vi "CIMAQ_Resample_Proportional.vi"(7 "Interpolation Type":u32(ring) items=["Zero Order", "Bi-Linear", "Quadratic", "Cubic Spline"], 8 "Error In":errorcluster, 9 "YResolution":u32, 10 "X Resolution":u32, 11 "Image In":T1) -> (0 "Error Out":errorcluster, 1 "Y Resolution":i32, 2 "X Resolution":i32, 3 "Image Out":T1)   [LabVIEW 2017]
uses:
  <vilib>/vision/Image Controls.llb/IMAQ Image.ctl
  <vilib>/vision/NI_Vision_Development_Module.lvlib
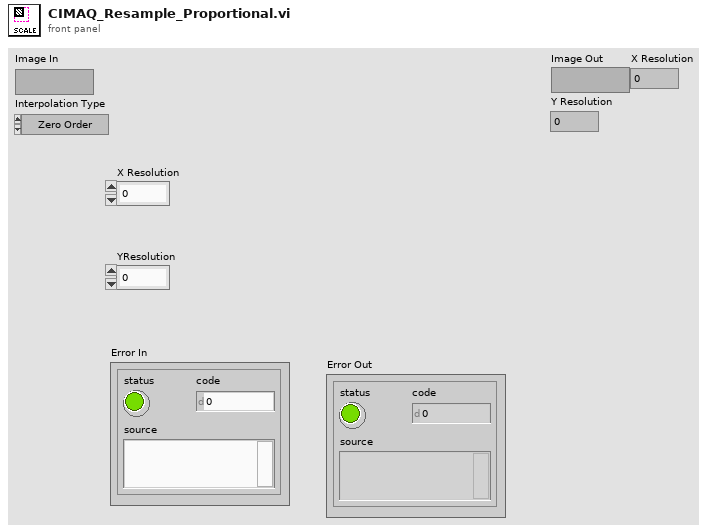
[diagram p1: front panel]
types:
  T1 = typedef "IMAQ Image.ctl" = refnum<image>
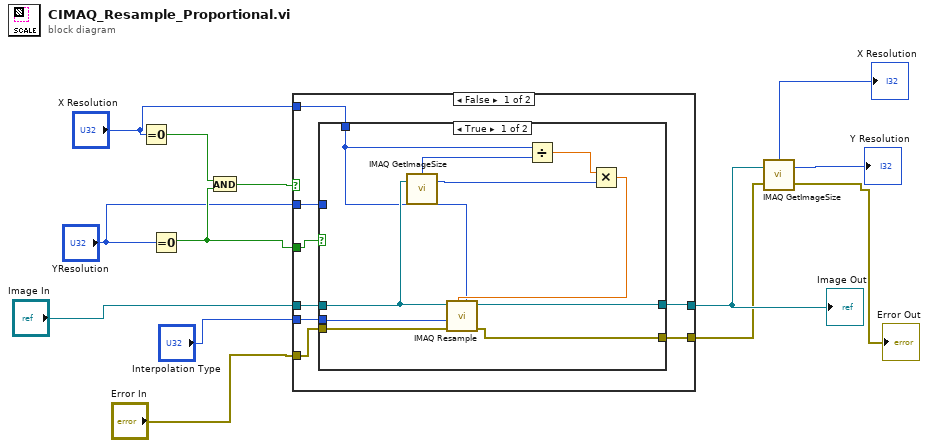
[diagram p0: block diagram]
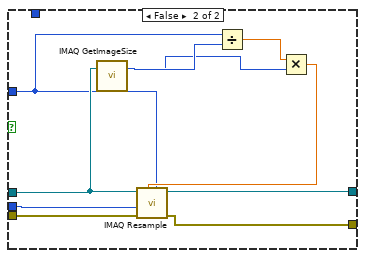
[diagram p2: hidden frame]
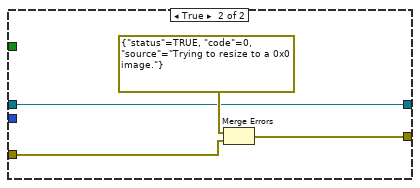
[diagram p3: hidden frame]
diagram:
  n1 = Equal To 0?(x="X Resolution") -> (x = 0?=w12:bool)
  n2 = Equal To 0?(x="YResolution") -> (x = 0?=w9:bool)
  n3 = And(x=w12, y=w9) -> (x .and. y?=w11:bool)
  n4 = case shown="False" w11 {
    tunnel: "Image In" -> [w21 w42]
    tunnel: "Error In" -> [w17 w45]
    tunnel: [w16 w43] -> w3
    tunnel: [w18 w42] -> w6
    tunnel: w9 -> [w20 _]
    tunnel: "X Resolution" -> [w19 _]
    tunnel: "YResolution" -> [w15 _]
    tunnel: "Interpolation Type" -> [w14 _]
    frame False {
      n5 = case shown="True" w20 {
        tunnel: w21 -> [w27 w39]
        tunnel: w19 -> [w26 _]
        tunnel: [w25 w38] -> w18
        tunnel: w17 -> [w24 w37]
        tunnel: [w23 w36] -> w16
        tunnel: w15 -> [_ w35]
        tunnel: w14 -> [w22 w32]
        frame True {
          n6 = call "IMAQ GetImageSize"("Image"=w27) -> ("Y Resolution"=w29:i32, "X Resolution"=w31:i32)  [unwired: 3 in, 1 out]
          n7 = Divide(x=w26, y=w31) -> (x/y=w30:dbl)
          n8 = Multiply(x=w30, y=w29) -> (x*y=w28:dbl)
          n9 = call "IMAQ Resample"("X Resolution"=w26, "Y Resolution"=w28, "error in (no error)"=w24, "Interpolation Type"=w22, "Image Src"=w27) -> ("error out"=w23:errorcluster, "Image Dst Out"=w25:T1)  [unwired: 5 in]
        }
        frame False {
          n10 = call "IMAQ GetImageSize"("Image"=w39) -> ("Y Resolution"=w34:i32, "X Resolution"=w33:i32)  [unwired: 3 in, 1 out]
          n11 = Divide(x=w35, y=w34) -> (x/y=w41:dbl)
          n12 = Multiply(x=w41, y=w33) -> (x*y=w40:dbl)
          n13 = call "IMAQ Resample"("X Resolution"=w35, "Y Resolution"=w40, "error in (no error)"=w37, "Interpolation Type"=w32, "Image Src"=w39) -> ("error out"=w36:errorcluster, "Image Dst Out"=w38:T1)  [unwired: 5 in]
        }
      }
    }
    frame True {
      n14 = Merge Errors(errorcluster {"status"=TRUE, "code"=0, "source"="Trying to resize to a 0x0 image."} ("error in"), w45) -> (w43:errorcluster)
    }
  }
  "Image Out" <- w6
  n15 = call "IMAQ GetImageSize"("Image"=w6, "error in (no error)"=w3) -> ("Y Resolution"=→"Y Resolution":i32, "X Resolution"=→"X Resolution":i32, "error out"=→"Error Out":errorcluster)  [unwired: 2 in]
